vi "global.vi"() -> ()   [LabVIEW 2019]
uses:
  System Monitor Cluster.ctl
panel:
  out "Stop Heat (s)":dbl
  out "Start Heat (s)":dbl
  out "Pules Height":dbl
  out "Lock In #3 Sensitivity":i32(ring)=19 items=["2 nV/fA", "5 nV/fA", "10 nV/fA", "20 nV/fA", "50 nV/fA", "100 nV/fA", "200 nV/fA", "500 nV/fA", "1 µV /pA", "2 µV/pA", "5 µV/pA", "10 µV/pA", "20 µV/pA", "50 µV/pA", "100 µV/pA", "200 µV/pA", "500 µV/pA", "1 mV/nA", "2 mV/nA", "5 mV/nA", "10 mV/nA", "20 mV/nA", "50 mV/nA", "100 mV/nA", "200 mV/nA", "500 mV/nA", "1 V/µA"]
  out "Measurement Running?":bool
  out "Sweep final rate":dbl
  out "Sweep init rate":dbl
  out "Step-Init":bool
  out "phi_final":dbl
  out "phi_init":dbl
  out "6221 Offset":dbl
  out "6221 Frequency":dbl
  out "6221 Current":dbl
  out "System Monitor Variables":T1={"Time"=[], "LI1CH1"=[], "LI1CH2"=[], "LI2CH1"=[], "LI2CH2"=[], "LI3CH1"=[], "LI3CH2"=[], "Field"=[], "N_Level"=[], "H_Level"=[], "Heat_370"=[], "Sorb_Heat"=[], "Still_Heat"=[], "Capacity"=[], "Loss"=[], "Magnet_Temperature"=[], "Lam_Pressure"=[], "Lam_NValve"=[], "370-T1"=[], "370-T2"=[], "370-T3"=[], "370-T4"=[], "370-T5"=[], "370-R1"=[], "370-R2"=[], "370-R3"=[], "370-R4"=[], "370-R5"=[], "372-T1"=[], "372-T2"=[], "372-T3"=[], "372-T4"=[], "372-T5"=[], "372-T6"=[], "372-R1"=[], "372-R2"=[], "372-R3"=[], "372-R4"=[], "372-R5"=[], "372-R6"=[], "Nada"=[nan], "K2440_Res"=[], "K2440_Current"=[], "VTI_Heater"=[], "VTI_NValve"=[], "LS340_Heater"=[], "K6221_Amplitude"=[], "K6221_Frequency"=[], "Cond_Pressure"=[], "Still_Pressure"=[], "FP_Out_Pressure"=[], "Dump_Pressure"=[], "V1"=[], "V2"=[], "V4"=[], "V5"=[], "V9"=[], "Forepump"=[], "Compressor"=[], "K6221_Offset"=[], "BoxTemp"=[], "By"=[], "Bz"=[], "Phi"=[], "heater-recond (%)"=[], "Dewar Pressure "=[], "JT-SP-Control"=[], "350 T1"=[], "350 T2"=[], "350 T3"=[], "350 T4"=[], "350 R1"=[], "350 R2"=[], "350 R3"=[], "350 R4"=[], "Angle"=[], "VTI CH1"=[], "VTI CH2"=[], "VTI CH3"=[], "ColdTrap"=[], "Mischer Pot"=[], "G1 (mbar)"=[], "G3 (mbar) "=[], "G4 (mbar)"=[], "IVC (mbar)"=[], "P2 (mbar) "=[], "Pot mischer (mbar)"=[], "AVS Control Channel (K)"=[], "AVS Control Channel (RES)"=[], "AVS  Channel 5 (RES) "=[], "LI3CH3"=[], "LI3CH4"=[], "LI1CH3"=[], "LI1CH4"=[], "LI2CH3"=[], "LI2CH4"=[], "Volt"=[], "Watt"=[], "Torque Angle"=[], "Dewar heater (W)"=[], "PSU Voltage"=[], "Turbopump"=[], "372-R7"=[], "372-T7"=[], "SIM921 Ch1"=[], " He3 Temp1"=[], " He3 Temp 2"=[], "LI4CH1"=[], "LI4CH2"=[]}
  out "Exponent":dbl
  out "Sweep Type":string
  out "Sweep final":dbl
  out "Sweep init":dbl
  out "Frequency":dbl
  out "Set JT Temperature Sweep":bool
  out "T-Loop (JT)":bool
  out "Angle  init. \nGeschw":dbl
  out "Angle final (Deg)":dbl
  out "Angle Geschw.":i32
  out "Angle  init.(Deg)":dbl
  out "-CC":dbl
  in  "Current Lakeshore Channel":dbl
  out "current I init 3":dbl
  out "current I init 2":dbl
  out "current I final":dbl
  out "number of steps in step sweep":i32
  out "current I init":dbl
  out "Needle Valve Value":dbl
  out "Needle Valve Constant?":i32
  out "Minutes to wait\nafter initialization":dbl
  out "Lock In #2 Sensitivity":i32(ring)=19 items=["2 nV/fA", "5 nV/fA", "10 nV/fA", "20 nV/fA", "50 nV/fA", "100 nV/fA", "200 nV/fA", "500 nV/fA", "1 µV /pA", "2 µV/pA", "5 µV/pA", "10 µV/pA", "20 µV/pA", "50 µV/pA", "100 µV/pA", "200 µV/pA", "500 µV/pA", "1 mV/nA", "2 mV/nA", "5 mV/nA", "10 mV/nA", "20 mV/nA", "50 mV/nA", "100 mV/nA", "200 mV/nA", "500 mV/nA", "1 V/µA"]
  out "Lock In #1 Sensitivity":i32(ring)=19 items=["2 nV/fA", "5 nV/fA", "10 nV/fA", "20 nV/fA", "50 nV/fA", "100 nV/fA", "200 nV/fA", "500 nV/fA", "1 µV /pA", "2 µV/pA", "5 µV/pA", "10 µV/pA", "20 µV/pA", "50 µV/pA", "100 µV/pA", "200 µV/pA", "500 µV/pA", "1 mV/nA", "2 mV/nA", "5 mV/nA", "10 mV/nA", "20 mV/nA", "50 mV/nA", "100 mV/nA", "200 mV/nA", "500 mV/nA", "1 V/µA"]
  out "Cerrent Measurement":i32(ring) items=["--", "resistance A", "resistance B", "resistance C", "magn. A", "magn. B", "magn. C"]
  out "Measurement 6":i32(ring) items=["--", "Lock In 1 - SR 830", "Lock In 2 - SR 830", "---", "----", "-----", "------"]
  out "Measurement 5":i32(ring) items=["--", "Lock In 1 - SR 830", "Lock In 2 - SR 830", "---", "----", "-----", "------"]
  out "Measurement 4":i32(ring) items=["--", "Lock In 1 - SR 830", "Lock In 2 - SR 830", "---", "----", "-----", "------"]
  out "Measurement 3":i32(ring) items=["--", "Lock In 1 - SR 830", "Lock In 2 - SR 830", "---", "----", "-----", "------"]
  out "Measurement 2":i32(ring) items=["--", "Lock In 1 - SR 830", "Lock In 2 - SR 830", "---", "----", "-----", "------"]
  out "Measurement 1":i32(ring) items=["--", "Lock In 1 - SR 830", "Lock In 2 - SR 830", "---", "----", "-----", "------"]
  out "-ter Messungsreihe":dbl
  out "H  init. \nGeschw.(T/min)":dbl
  out "T  init. Geschw. \n(K/min)":dbl
  out "Cerrent State":i32(ring) items=["--", "Initial", "CS Schleife", "SC Schleife", "CC Schleife", "CS-Step", "I-sweep"]
  out "Env.":i32
  out "H final (T)":dbl
  out "H Geschw.(T/min)":dbl
  out "H init.(T)":dbl
  out "T final (K)":dbl
  out "T Geschw. \n(K/min)":dbl
  out "T init. (K)":dbl
  out "Control Array":dbl[][](array[numeric])
  # "AMI Phi (Deg)"
  # "aktuelle\nMessungsreihe"
  # "Control Array"
  # "AH Frequency"
  # "Channel nuber Ls370"
  # "current I final"
  # "N.V. Constant?"
  # "Env0"
  # "T init"
  # "T init \nGeschw."
  # "T final"
  # "T final \nGeschw."
  # "H init"
  # "H init \nGeschw."
  # "H final"
  # "H final \nGeschw."
  # "LI#1 Sens"
  # "LI#2 Sens"
  # "LI#3 Sens"
  # "6221c"
  # "6221f"
  # "Angle fin"
  # "6221off"
  # "Angle init"
  # "wait"
  # "N.V. Value"
  # "# Steps"
  # "current I init"
  # "Current Measurement\nwithin CC-loop"
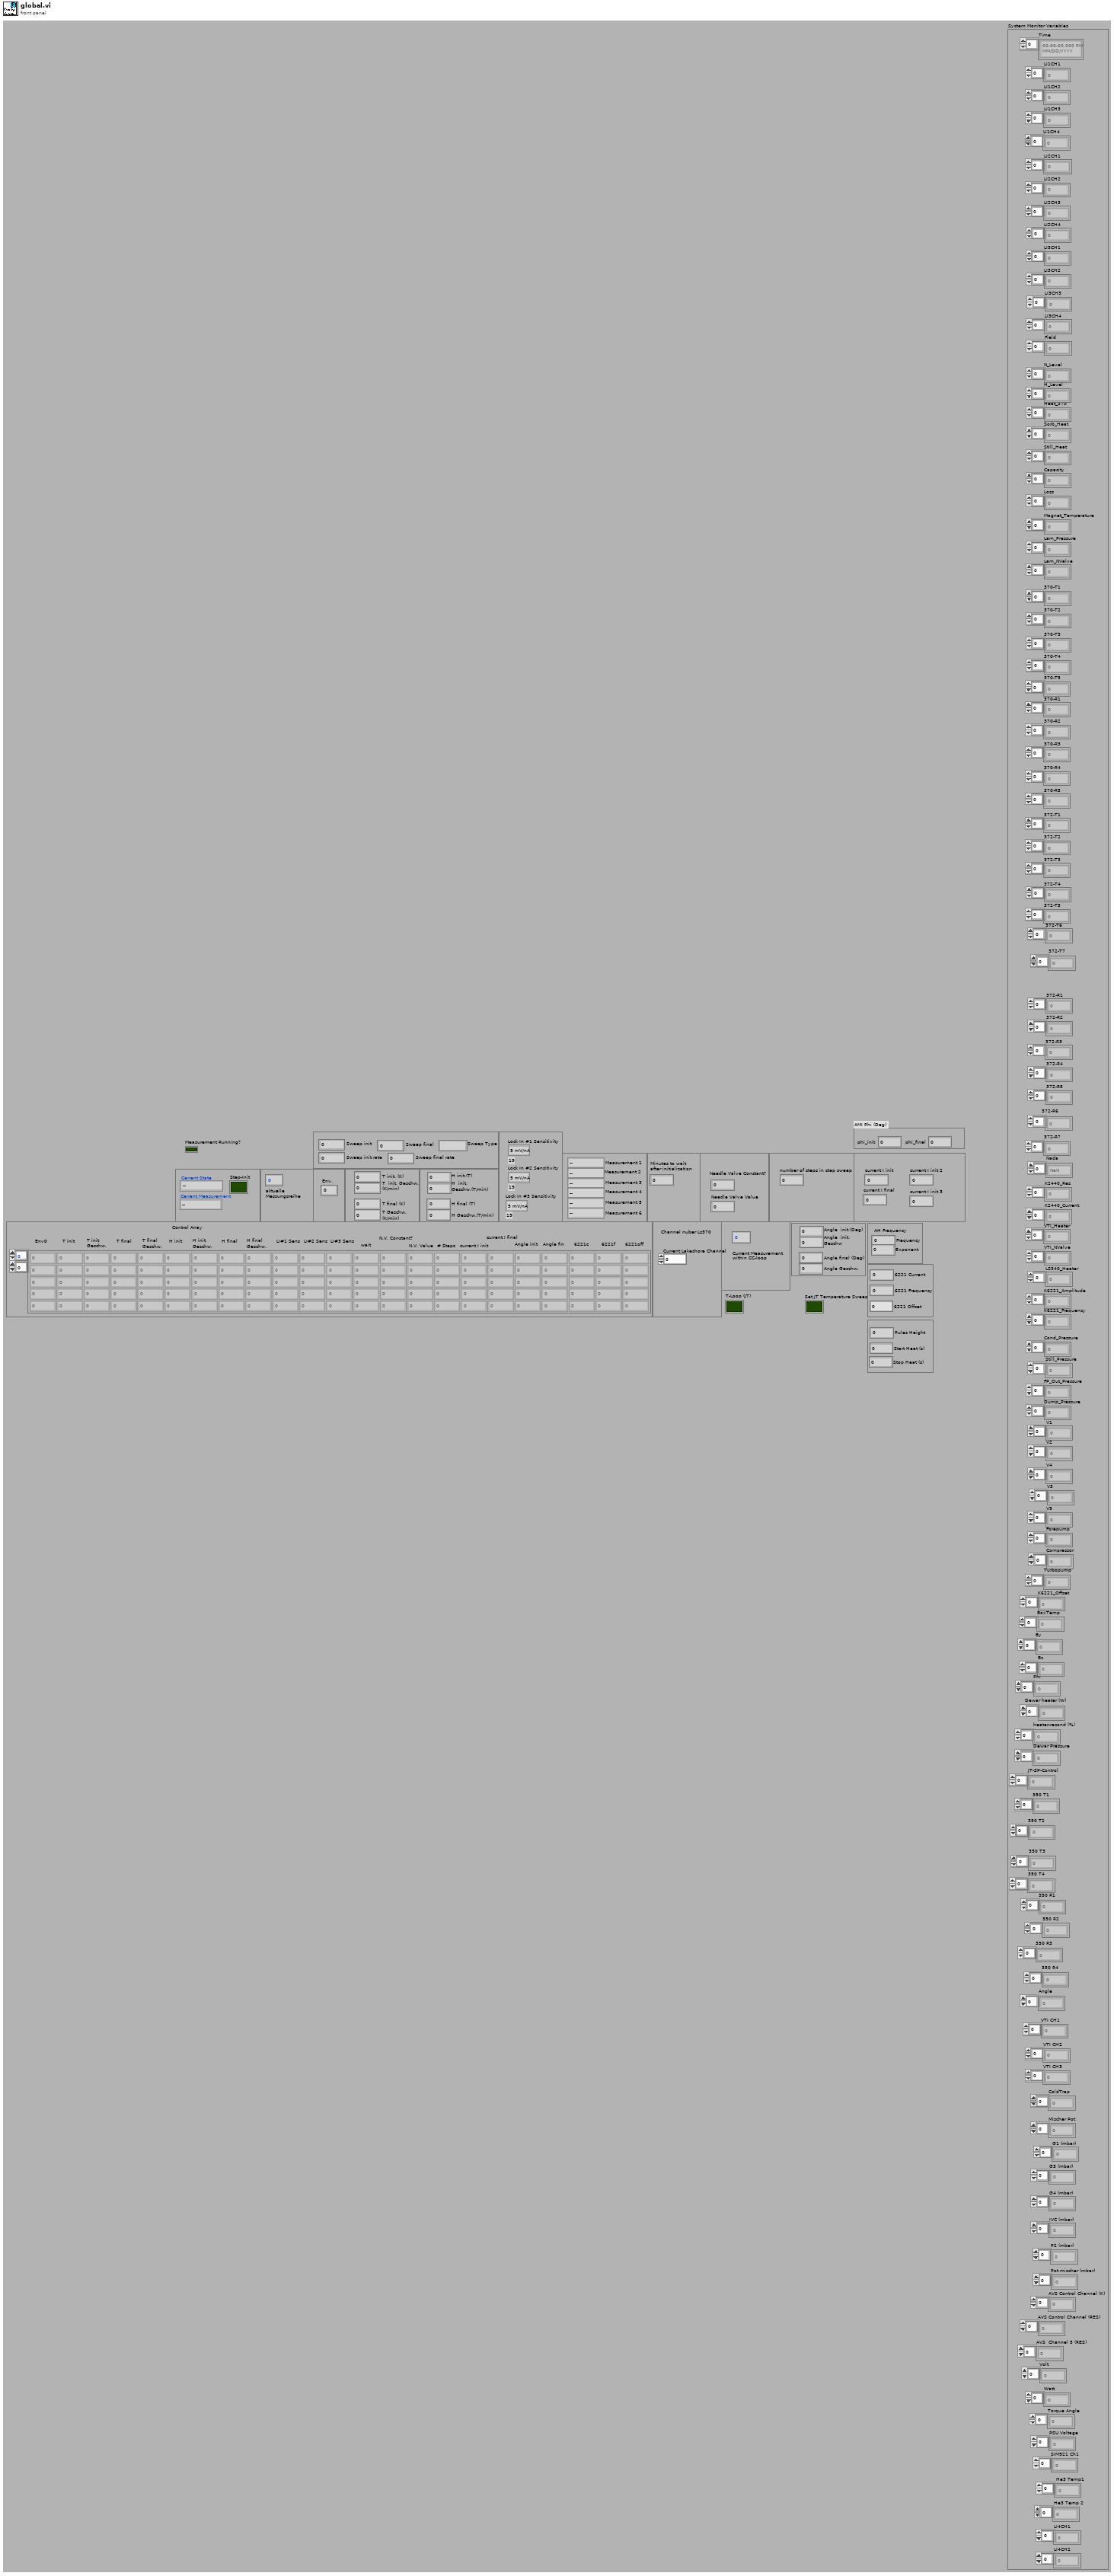
[diagram p1: front panel]
types:
  T1 = typedef "System Monitor Cluster.ctl" = cluster{"Time":timestamp[], "LI1CH1":dbl[], "LI1CH2":dbl[], "LI2CH1":dbl[], "LI2CH2":dbl[], "LI3CH1":dbl[], "LI3CH2":dbl[], "Field":dbl[], "N_Level":dbl[], "H_Level":dbl[], "Heat_370":dbl[], "Sorb_Heat":dbl[], "Still_Heat":dbl[], "Capacity":dbl[], "Loss":dbl[], "Magnet_Temperature":dbl[], "Lam_Pressure":dbl[], "Lam_NValve":dbl[], "370-T1":dbl[], "370-T2":dbl[], "370-T3":dbl[], "370-T4":dbl[], "370-T5":dbl[], "370-R1":dbl[], "370-R2":dbl[], "370-R3":dbl[], "370-R4":dbl[], "370-R5":dbl[], "372-T1":dbl[], "372-T2":dbl[], "372-T3":dbl[], "372-T4":dbl[], "372-T5":dbl[], "372-T6":dbl[], "372-R1":dbl[], "372-R2":dbl[], "372-R3":dbl[], "372-R4":dbl[], "372-R5":dbl[], "372-R6":dbl[], "Nada":dbl[], "K2440_Res":dbl[], "K2440_Current":dbl[], "VTI_Heater":dbl[], "VTI_NValve":dbl[], "LS340_Heater":dbl[], "K6221_Amplitude":dbl[], "K6221_Frequency":dbl[], "Cond_Pressure":dbl[], "Still_Pressure":dbl[], "FP_Out_Pressure":dbl[], "Dump_Pressure":dbl[], "V1":dbl[], "V2":dbl[], "V4":dbl[], "V5":dbl[], "V9":dbl[], "Forepump":dbl[], "Compressor":dbl[], "K6221_Offset":dbl[], "BoxTemp":dbl[], "By":dbl[], "Bz":dbl[], "Phi":dbl[], "heater-recond (%)":dbl[], "Dewar Pressure ":dbl[], "JT-SP-Control":dbl[], "350 T1":dbl[], "350 T2":dbl[], "350 T3":dbl[], "350 T4":dbl[], "350 R1":dbl[], "350 R2":dbl[], "350 R3":dbl[], "350 R4":dbl[], "Angle":dbl[], "VTI CH1":dbl[], "VTI CH2":dbl[], "VTI CH3":dbl[], "ColdTrap":dbl[], "Mischer Pot":dbl[], "G1 (mbar)":dbl[], "G3 (mbar) ":dbl[], "G4 (mbar)":dbl[], "IVC (mbar)":dbl[], "P2 (mbar) ":dbl[], "Pot mischer (mbar)":dbl[], "AVS Control Channel (K)":dbl[], "AVS Control Channel (RES)":dbl[], "AVS  Channel 5 (RES) ":dbl[], "LI3CH3":dbl[], "LI3CH4":dbl[], "LI1CH3":dbl[], "LI1CH4":dbl[], "LI2CH3":dbl[], "LI2CH4":dbl[], "Volt":dbl[], "Watt":dbl[], "Torque Angle":dbl[], "Dewar heater (W)":dbl[], "PSU Voltage":dbl[], "Turbopump":dbl[], "372-R7":dbl[], "372-T7":dbl[], "SIM921 Ch1":dbl[], " He3 Temp1":dbl[], " He3 Temp 2":dbl[], "LI4CH1":dbl[], "LI4CH2":dbl[]}
diagram:
